vi "Get Ingredients.vi"(8 "error in (no error)":errorcluster, 11 "Circuit Board in":refnum<class "Circuit Board.lvclass">) -> (0 "error out":errorcluster, 2 "Ingredients":T1[](array[typedef]), 3 "Circuit Board out":refnum<class "Circuit Board.lvclass">)   [LabVIEW 2020, in "Circuit Board.lvclass"]
uses:
  Circuit Board.lvclass
  Item/Ingredient.ctl
  Item/Item.lvclass
  Metal/Metal.lvclass
  C:/dev/LabVIEW/Good Company Calc/Item/Item.lvclass
  Plastic/Plastic.lvclass
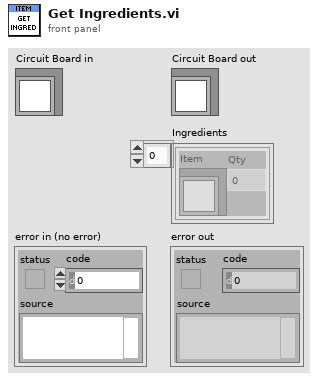
[diagram p1: front panel]
types:
  T1 = typedef "Item.lvclass/Ingredient.ctl" = cluster{"Item":refnum<class "Item.lvclass">, "Qty":dbl}
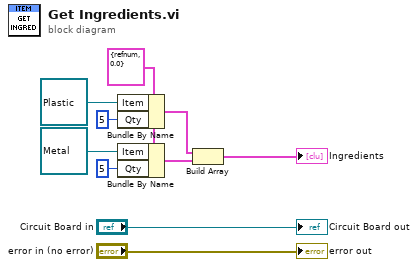
[diagram p0: block diagram]
diagram:
  w5 = T1 {"Item"=refnum, "Qty"=0.0} ("Ingredient")
  n1 = Bundle By Name(cluster=w5, "Item"=refnum<class "Plastic.lvclass"> refnum ("Plastic.lvclass"), "Qty"=5) -> (w3:T1)
  n2 = Bundle By Name(cluster=w5, "Item"=refnum<class "Metal.lvclass"> refnum ("Metal.lvclass"), "Qty"=5) -> (w4:T1)
  n3 = Build Array(w3, w4) -> (→"Ingredients":T1[])
  "error out" <- "error in (no error)"
  "Circuit Board out" <- "Circuit Board in"
